vi "pulmonarytesting_pressurediameterlogging.vi"() -> ()   [LabVIEW 2014]
uses:
  <vilib>/vision/NI_Vision_Development_Module.lvlib
  <instrlib>/KD Scientific 2XX Series/KD Scientific 2XX Series.lvlib
panel:
  in  "stop 4":bool
  in  "Baud Rate (9600)":u32(ring)=9600 items=["300"=300, "1200"=1200, "2400"=2400, "4800"=4800, "9600"=9600]
  in  "Withdrawal Settings":T1={"Flow Rate (5)"=5.0, "Volume (10)"=10.0, "Volume Units (ml)"=enum."milliliters (ml)", "Rate Units (ml/min.)"=enum."milliliters per minute (ml/min.)"} {"Volume (10)" format="%#.3g"}
  in  "Diameter (8.75 mm)":dbl=8.75
  in  "Infusion Settings":T1={"Flow Rate (5)"=5.0, "Volume (10)"=10.0, "Volume Units (ml)"=enum."milliliters (ml)", "Rate Units (ml/min.)"=enum."milliliters per minute (ml/min.)"}
  out "Status":T2
  in  "stop 2":bool
  out "Delivered Volume":dbl
  out "Units":string
  in  "Operation Mode (Infuse)":u16(ring) items=["Infuse", "Withdraw", "Infuse-Withdraw", "Withdraw-Infuse", "Continuous"]
  in  "Address (0)":i32 format="%0.0f"
  in  "error in (no error)":errorcluster
  in  "VISA resource name":refnum<visa-resource-name>="COM1"
  in  "stop":bool
  out "Image":T3(plugin-control)
  out "Particle Measurements (Pixels) (Particle Analysis 1)":dbl[][](array[numeric]) format="%.2f"
  out "subarray":dbl[](array[numeric])
  out "The diameter":dbl[](array[numeric])
  in  "stop (F)":bool
  out "Data from Transducer":dynamicdata(graph) caption="Voltage from Transducer V"
  out "Voltage from pressure transducer":dbl[](array[numeric])
  out "Pressure mm Hg":dbl[](graph)
  in  "Calibration factor":dbl[](array[numeric])
  in  "Zero Error":dbl[](array[numeric])
  out "pressure mm Hg":dbl[](array[numeric])
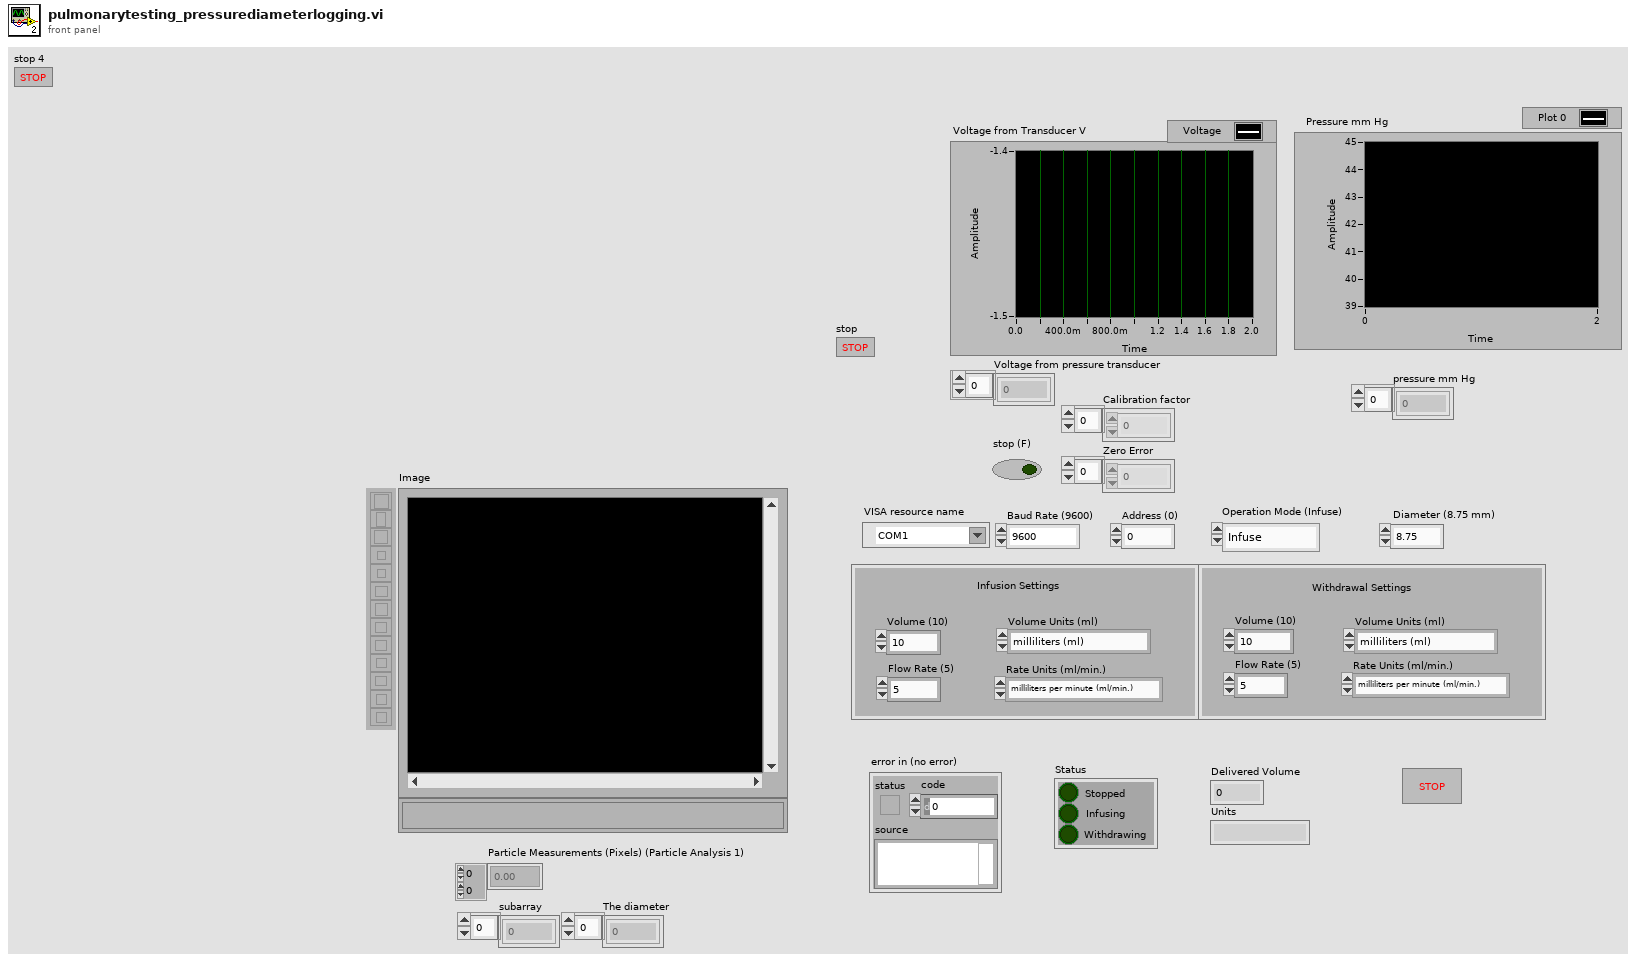
[diagram p1: front panel]
types:
  T1 = cluster{"Flow Rate (5)":dbl, "Volume (10)":dbl, "Volume Units (ml)":enum16{"milliliters (ml)", "microliters (ul)"}, "Rate Units (ml/min.)":enum16{"milliliters per minute (ml/min.)", "milliliters per hour (ml/hr.)", "microliters per minute (ul/min.)", "microliters per hour (ul/hr.)"}}
  T2 = cluster{"Stopped":bool, "Infusing":bool, "Withdrawing":bool}
  T3 = typedef "IMAQ Image.ctl" = refnum<image>
  T4 = typedef "Board Id" = u8
  T5 = typedef "ROI Descriptor" = cluster{"Global Rectangle":i32[], "Contours":cluster{"ID":enum32{"External", "Internal"}, "Type":u32, "Coordinates":i32[]}[]}
  T6 = enum16{"milliliters per minute (ml/min.)", "milliliters per hour (ml/hr.)", "microliters per minute (ul/min.)", "microliters per hour (ul/hr.)"}
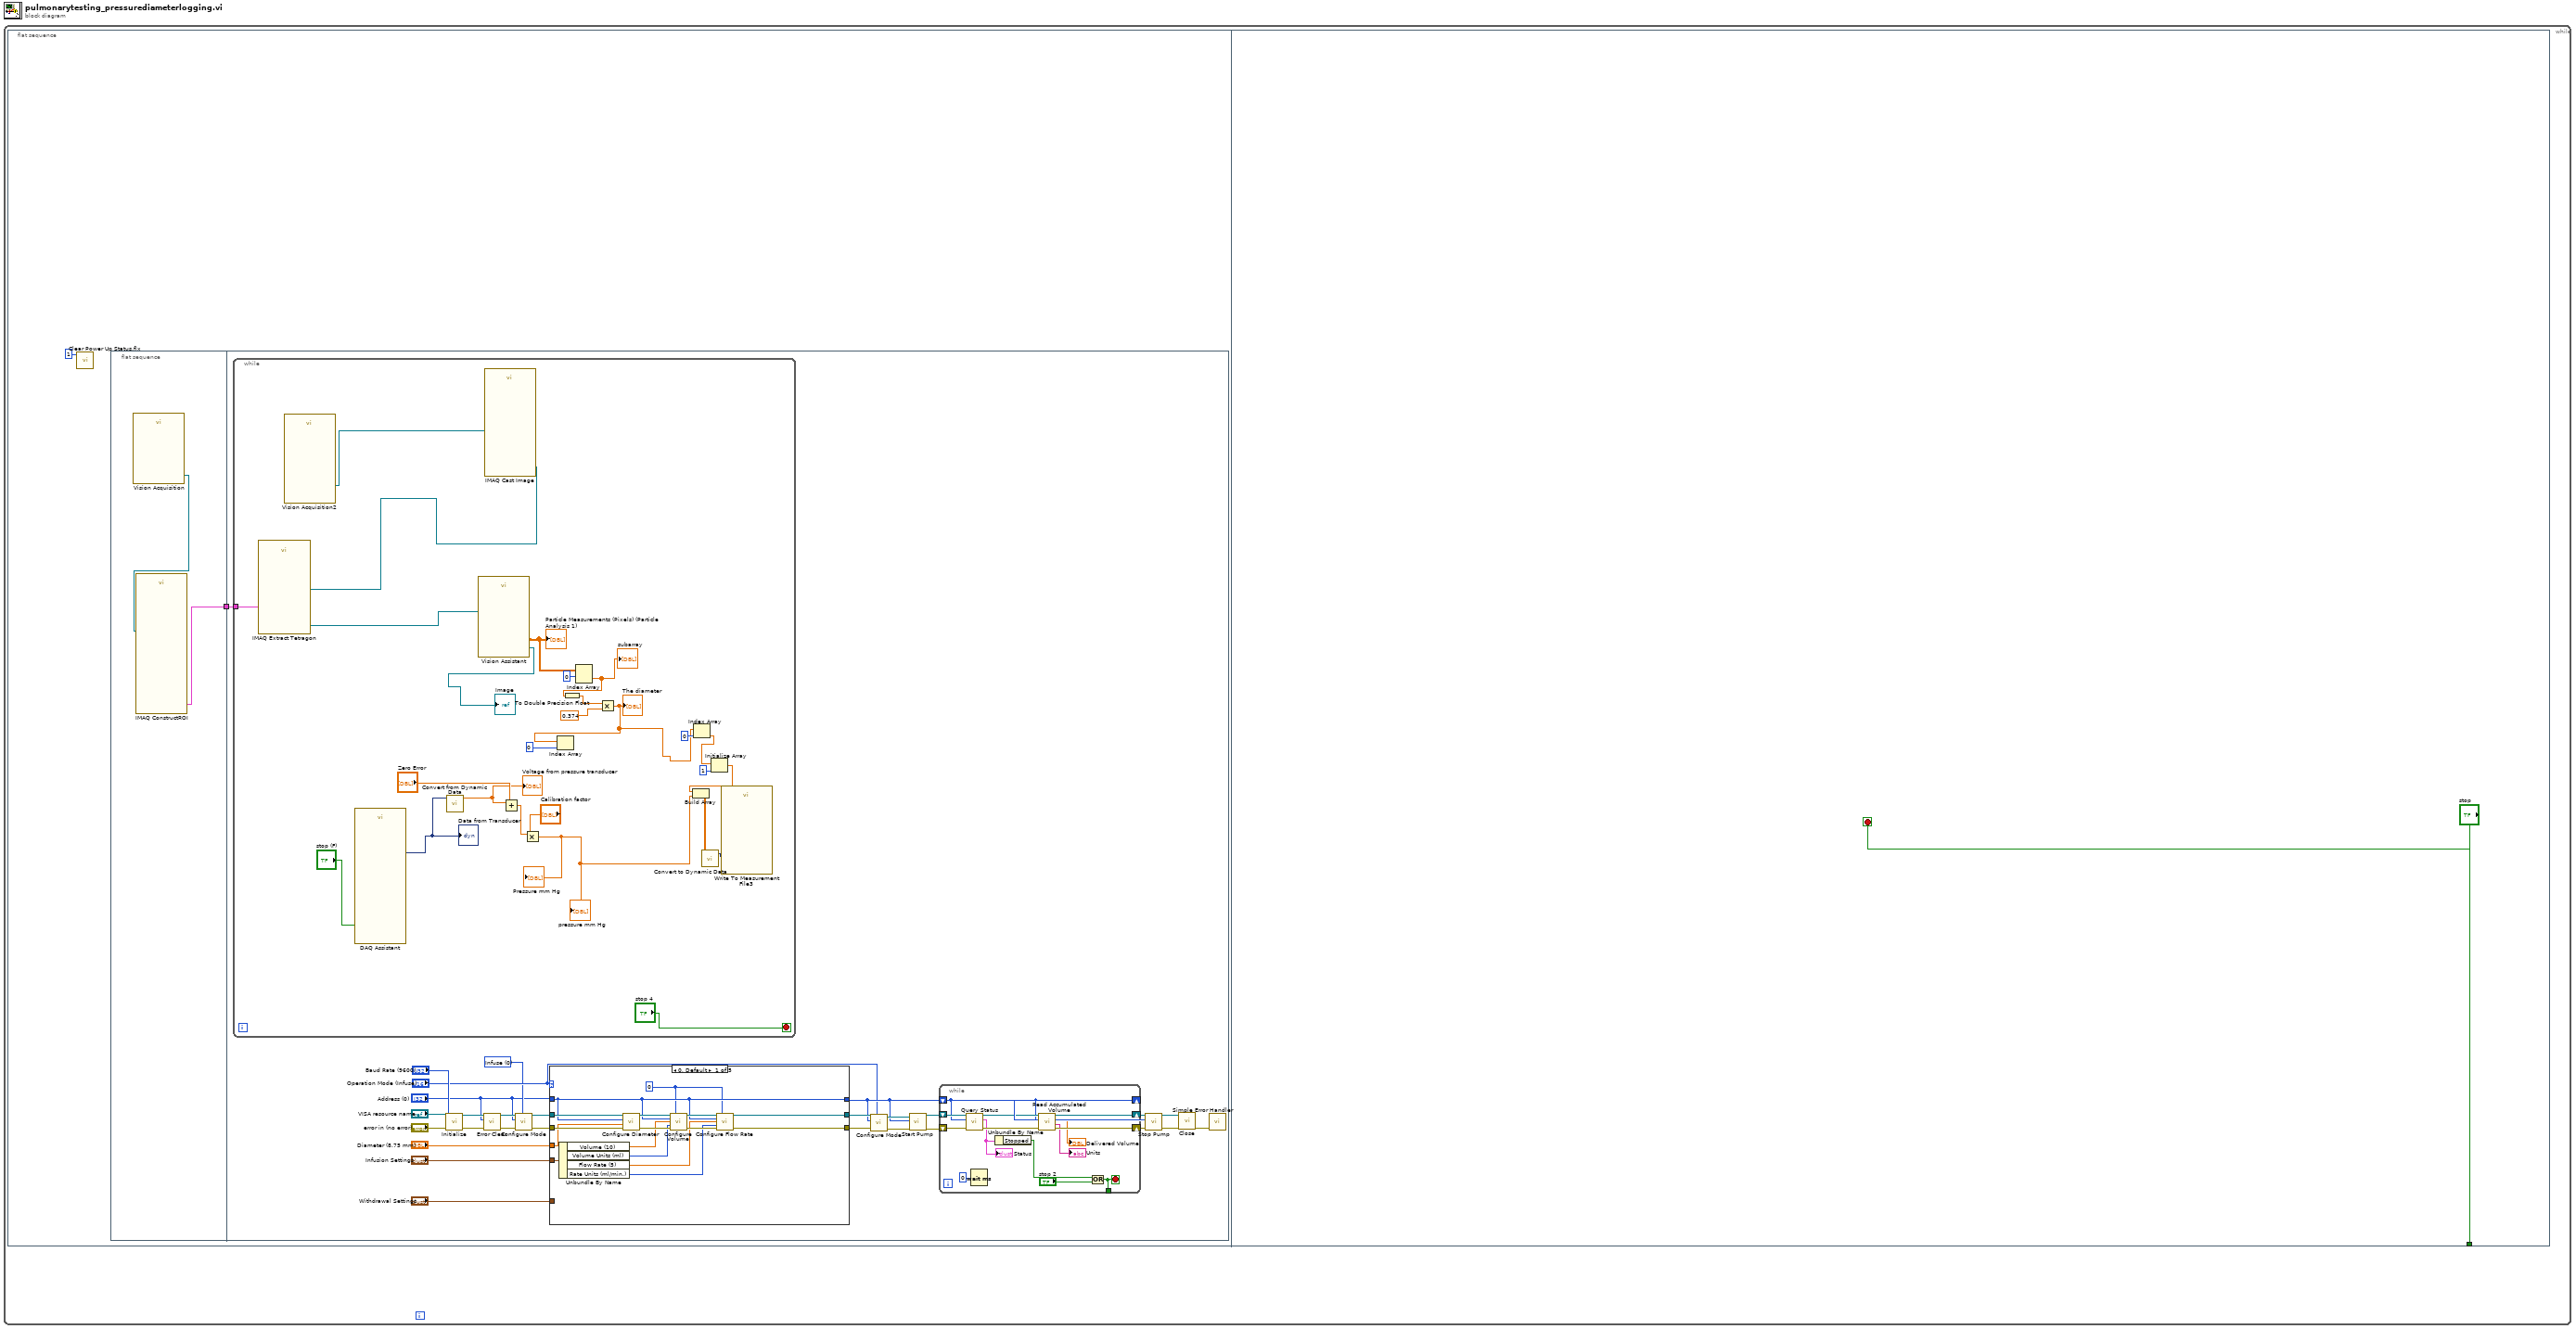
[diagram p0: block diagram]
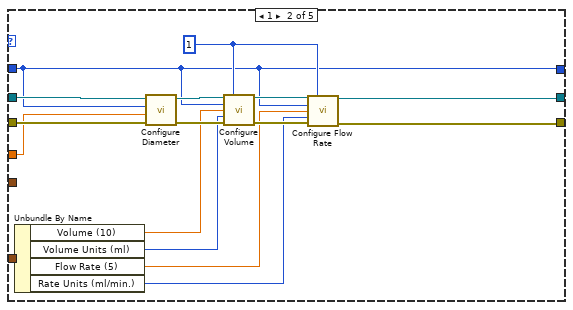
[diagram p2: hidden frame]
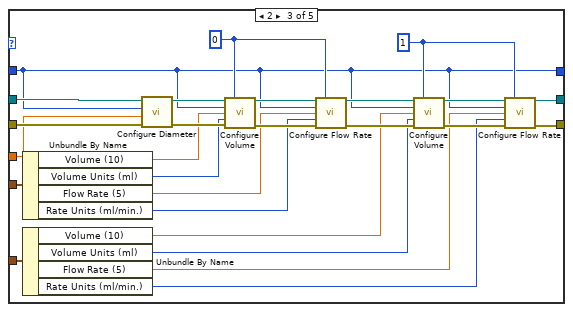
[diagram p3: hidden frame]
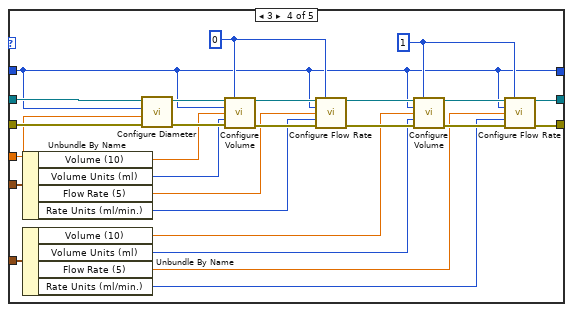
[diagram p4: hidden frame]
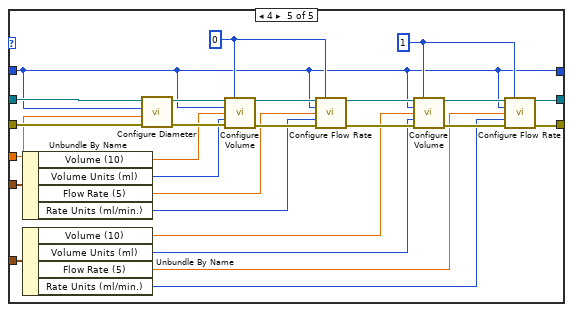
[diagram p5: hidden frame]
diagram:
  n1 = while {
    stop <- w1 stop-if-true
    n2 = flat-sequence {
      tunnel: ["stop"] -> w1
      frame #0 {
        n3 = call <vilib>:"Clear Power Up Status.flx"("Board ID"=T4 1) -> ()  [unwired: 6 in, 2 out]
        n4 = flat-sequence {
          tunnel: [w4] -> w3
          tunnel: w3 -> [w34]
          frame #0 {
            n5 = call "Vision Acquisition"() -> ("Image Out"=w5:T3)  [unwired: 26 in, 1 out]
            n6 = call "IMAQ ConstructROI"("Image"=w5) -> ("ROI Descriptor Out"=w4:T5)  [unwired: 7 in, 3 out]
          }
          frame #1 {
            w11 = u16 0 items=["Infuse", "Withdraw", "Infuse-Withdraw", "Withdraw-Infuse", "Continuous"] ("Mode (infuse)")
            n7 = while {
              tunnel: w34 -> [w60]
              stop <- "stop 4" stop-if-true
              n8 = call "Vision Acquisition2"() -> ("Image Out"=w44:T3)  [unwired: 25 in, 2 out]
              n9 = call "DAQ Assistant"("stop (F)"="stop (F)") -> ("data"=w59:dynamicdata)  [unwired: 15 in, 3 out]
              "Data from Transducer" <- w59
              n10 = call "Convert from Dynamic Data"("Dynamic Data Type"=w59) -> ("Array"=w56:dbl[])  [unwired: 3 in]
              "Voltage from pressure transducer" <- w56
              n11 = call "IMAQ Cast Image"("Image Src"=w44) -> ("Image Dst Out"=w51:T3)  [unwired: 9 in, 1 out]
              n12 = call-poly "IMAQ Extract Tetragon"("ROI Descriptor"=w60, "Image Src"=w51) -> ("Image Dst Out"=w52:T3)  [unwired: 8 in, 1 out]
              n13 = call "Vision Assistant"("Image In"=w52) -> ("Image Out"=→"Image":T3, "Particle Measurements (Pixels) (Particle Analysis 1)"=w50:dbl[][])  [unwired: 23 in, 2 out]
              "Particle Measurements (Pixels) (Particle Analysis 1)" <- w50
              n14 = Add(x=w56, y="Zero Error") -> (x+y=w58:dbl[])
              n15 = Multiply(x=w58, y="Calibration factor") -> (x*y=w42:dbl[])
              "Pressure mm Hg" <- w42
              "pressure mm Hg" <- w42
              n16 = Index Array(array=w50, index (row)=0) -> (element=w48:dbl[])  [unwired: 1 in]
              "subarray" <- w48
              n17 = To Double Precision Float(number=w48) -> (double precision float=w47:dbl[])
              n18 = Multiply(x=w47, y=0.374) -> (x*y=w40:dbl[])
              "The diameter" <- w40
              n19 = Index Array(array=w40, index=0) -> ()  [unwired: 1 out]
              n20 = Index Array(array=w40, index=0) -> (element=w39:dbl)
              n21 = Initialize Array(w39, 1 ("dimension size")) -> (w37:dbl[])
              n22 = Build Array(w37, w42) -> (w36:dbl[][])
              n23 = call "Convert to Dynamic Data"("2D Array"=w36) -> ("Dynamic Data Type"=w35:dynamicdata)  [unwired: 3 in]
              n24 = call "Write To Measurement File3"("Signals"=w35) -> ()  [unwired: 16 in, 3 out]
            }
            n25 = call <instrlib>:"Initialize.vi"("error in (no error)"="error in (no error)", "Baud Rate (9600)"="Baud Rate (9600)", "VISA resource name"="VISA resource name") -> ("error out"=w8:errorcluster, "VISA resource name out"=w7:refnum<visa-resource-name>)  [unwired: 7 in]
            n26 = call <instrlib>:"Error Clear.vi"("error in (no error)"=w8, "Address (0)"="Address (0)", "VISA resource name"=w7) -> ("error out"=w9:errorcluster, "VISA resource name out"=w10:refnum<visa-resource-name>)  [unwired: 6 in, 1 out]
            n27 = call <instrlib>:"Configure Mode.vi"("Mode (infuse)"=w11, "error in (no error)"=w9, "Address (0)"="Address (0)", "VISA resource name"=w10) -> ("error out"=w13:errorcluster, "VISA resource name out"=w12:refnum<visa-resource-name>)  [unwired: 6 in]
            n28 = case shown="0, Default" "Operation Mode (Infuse)" {
              tunnel: "Infusion Settings" -> [w70 _ w118 w144 w170]
              tunnel: "Withdrawal Settings" -> [_ w92 w117 w143 w169]
              tunnel: w12 -> [w76 w91 w116 w142 w168]
              tunnel: w13 -> [w75 w87 w115 w141 w167]
              tunnel: "Diameter (8.75 mm)" -> [w69 w83 w98 w124 w150]
              tunnel: [w68 w77 w93 w119 w145] -> w15
              tunnel: "Address (0)" -> [w68 w77 w93 w119 w145]
              tunnel: [w63 w88 w95 w121 w147] -> w19
              tunnel: [w62 w84 w94 w120 w146] -> w18
              frame 0, Default {
                w61 = 0
                n29 = Unbundle By Name(w70) -> ("Volume (10)"=w67:dbl, "Volume Units (ml)"=w66:enum16{"milliliters (ml)", "microliters (ul)"}, "Flow Rate (5)"=w65:dbl, "Rate Units (ml/min.)"=w64:T6)
                n30 = call <instrlib>:"Configure Diameter.vi"("error in (no error)"=w75, "Diameter (8.75 mm)"=w69, "Address (0)"=w68, "VISA resource name"=w76) -> ("error out"=w73:errorcluster, "VISA resource name out"=w74:refnum<visa-resource-name>)  [unwired: 6 in]
                n31 = call <instrlib>:"Configure Volume.vi"("VISA resource name"=w74, "Mode (infuse)"=w61, "Address (0)"=w68, "Volume (100)"=w67, "Units (0: milliliters)"=w66, "error in (no error)"=w73) -> ("VISA resource name out"=w72:refnum<visa-resource-name>, "error out"=w71:errorcluster)  [unwired: 8 in]
                n32 = call <instrlib>:"Configure Flow Rate.vi"("VISA resource name"=w72, "Mode (infuse)"=w61, "Address (0)"=w68, "Flow Rate (5)"=w65, "Units (0: milliliters per minute)"=w64, "error in (no error)"=w71) -> ("VISA resource name out"=w63:refnum<visa-resource-name>, "error out"=w62:errorcluster)  [unwired: 8 in]
              }
              frame 1 {
                w78 = 1
                n33 = Unbundle By Name(w92) -> ("Volume (10)"=w82:dbl, "Volume Units (ml)"=w81:enum16{"milliliters (ml)", "microliters (ul)"}, "Flow Rate (5)"=w80:dbl, "Rate Units (ml/min.)"=w79:T6)
                n34 = call <instrlib>:"Configure Diameter.vi"("error in (no error)"=w87, "Diameter (8.75 mm)"=w83, "Address (0)"=w77, "VISA resource name"=w91) -> ("error out"=w86:errorcluster, "VISA resource name out"=w90:refnum<visa-resource-name>)  [unwired: 6 in]
                n35 = call <instrlib>:"Configure Volume.vi"("VISA resource name"=w90, "Mode (infuse)"=w78, "Address (0)"=w77, "Volume (100)"=w82, "Units (0: milliliters)"=w81, "error in (no error)"=w86) -> ("VISA resource name out"=w89:refnum<visa-resource-name>, "error out"=w85:errorcluster)  [unwired: 8 in]
                n36 = call <instrlib>:"Configure Flow Rate.vi"("VISA resource name"=w89, "Mode (infuse)"=w78, "Address (0)"=w77, "Flow Rate (5)"=w80, "Units (0: milliliters per minute)"=w79, "error in (no error)"=w85) -> ("VISA resource name out"=w88:refnum<visa-resource-name>, "error out"=w84:errorcluster)  [unwired: 8 in]
              }
              frame 2 {
                w96 = 1
                w97 = 0
                n37 = Unbundle By Name(w118) -> ("Volume (10)"=w106:dbl, "Volume Units (ml)"=w105:enum16{"milliliters (ml)", "microliters (ul)"}, "Flow Rate (5)"=w104:dbl, "Rate Units (ml/min.)"=w103:T6)
                n38 = Unbundle By Name(w117) -> ("Volume (10)"=w102:dbl, "Volume Units (ml)"=w101:enum16{"milliliters (ml)", "microliters (ul)"}, "Flow Rate (5)"=w100:dbl, "Rate Units (ml/min.)"=w99:T6)
                n39 = call <instrlib>:"Configure Diameter.vi"("error in (no error)"=w115, "Diameter (8.75 mm)"=w98, "Address (0)"=w93, "VISA resource name"=w116) -> ("error out"=w110:errorcluster, "VISA resource name out"=w114:refnum<visa-resource-name>)  [unwired: 6 in]
                n40 = call <instrlib>:"Configure Volume.vi"("VISA resource name"=w114, "Mode (infuse)"=w97, "Address (0)"=w93, "Volume (100)"=w106, "Units (0: milliliters)"=w105, "error in (no error)"=w110) -> ("VISA resource name out"=w113:refnum<visa-resource-name>, "error out"=w109:errorcluster)  [unwired: 8 in]
                n41 = call <instrlib>:"Configure Flow Rate.vi"("VISA resource name"=w113, "Mode (infuse)"=w97, "Address (0)"=w93, "Flow Rate (5)"=w104, "Units (0: milliliters per minute)"=w103, "error in (no error)"=w109) -> ("VISA resource name out"=w112:refnum<visa-resource-name>, "error out"=w108:errorcluster)  [unwired: 8 in]
                n42 = call <instrlib>:"Configure Volume.vi"("VISA resource name"=w112, "Mode (infuse)"=w96, "Address (0)"=w93, "Volume (100)"=w102, "Units (0: milliliters)"=w101, "error in (no error)"=w108) -> ("VISA resource name out"=w111:refnum<visa-resource-name>, "error out"=w107:errorcluster)  [unwired: 8 in]
                n43 = call <instrlib>:"Configure Flow Rate.vi"("VISA resource name"=w111, "Mode (infuse)"=w96, "Address (0)"=w93, "Flow Rate (5)"=w100, "Units (0: milliliters per minute)"=w99, "error in (no error)"=w107) -> ("VISA resource name out"=w95:refnum<visa-resource-name>, "error out"=w94:errorcluster)  [unwired: 8 in]
              }
              frame 3 {
                w122 = 1
                w123 = 0
                n44 = Unbundle By Name(w144) -> ("Volume (10)"=w132:dbl, "Volume Units (ml)"=w131:enum16{"milliliters (ml)", "microliters (ul)"}, "Flow Rate (5)"=w130:dbl, "Rate Units (ml/min.)"=w129:T6)
                n45 = Unbundle By Name(w143) -> ("Volume (10)"=w128:dbl, "Volume Units (ml)"=w127:enum16{"milliliters (ml)", "microliters (ul)"}, "Flow Rate (5)"=w126:dbl, "Rate Units (ml/min.)"=w125:T6)
                n46 = call <instrlib>:"Configure Diameter.vi"("error in (no error)"=w141, "Diameter (8.75 mm)"=w124, "Address (0)"=w119, "VISA resource name"=w142) -> ("error out"=w136:errorcluster, "VISA resource name out"=w140:refnum<visa-resource-name>)  [unwired: 6 in]
                n47 = call <instrlib>:"Configure Volume.vi"("VISA resource name"=w140, "Mode (infuse)"=w123, "Address (0)"=w119, "Volume (100)"=w132, "Units (0: milliliters)"=w131, "error in (no error)"=w136) -> ("VISA resource name out"=w139:refnum<visa-resource-name>, "error out"=w135:errorcluster)  [unwired: 8 in]
                n48 = call <instrlib>:"Configure Flow Rate.vi"("VISA resource name"=w139, "Mode (infuse)"=w123, "Address (0)"=w119, "Flow Rate (5)"=w130, "Units (0: milliliters per minute)"=w129, "error in (no error)"=w135) -> ("VISA resource name out"=w138:refnum<visa-resource-name>, "error out"=w134:errorcluster)  [unwired: 8 in]
                n49 = call <instrlib>:"Configure Volume.vi"("VISA resource name"=w138, "Mode (infuse)"=w122, "Address (0)"=w119, "Volume (100)"=w128, "Units (0: milliliters)"=w127, "error in (no error)"=w134) -> ("VISA resource name out"=w137:refnum<visa-resource-name>, "error out"=w133:errorcluster)  [unwired: 8 in]
                n50 = call <instrlib>:"Configure Flow Rate.vi"("VISA resource name"=w137, "Mode (infuse)"=w122, "Address (0)"=w119, "Flow Rate (5)"=w126, "Units (0: milliliters per minute)"=w125, "error in (no error)"=w133) -> ("VISA resource name out"=w121:refnum<visa-resource-name>, "error out"=w120:errorcluster)  [unwired: 8 in]
              }
              frame 4 {
                w148 = 1
                w149 = 0
                n51 = Unbundle By Name(w170) -> ("Volume (10)"=w158:dbl, "Volume Units (ml)"=w157:enum16{"milliliters (ml)", "microliters (ul)"}, "Flow Rate (5)"=w156:dbl, "Rate Units (ml/min.)"=w155:T6)
                n52 = Unbundle By Name(w169) -> ("Volume (10)"=w154:dbl, "Volume Units (ml)"=w153:enum16{"milliliters (ml)", "microliters (ul)"}, "Flow Rate (5)"=w152:dbl, "Rate Units (ml/min.)"=w151:T6)
                n53 = call <instrlib>:"Configure Diameter.vi"("error in (no error)"=w167, "Diameter (8.75 mm)"=w150, "Address (0)"=w145, "VISA resource name"=w168) -> ("error out"=w162:errorcluster, "VISA resource name out"=w166:refnum<visa-resource-name>)  [unwired: 6 in]
                n54 = call <instrlib>:"Configure Volume.vi"("VISA resource name"=w166, "Mode (infuse)"=w149, "Address (0)"=w145, "Volume (100)"=w158, "Units (0: milliliters)"=w157, "error in (no error)"=w162) -> ("VISA resource name out"=w165:refnum<visa-resource-name>, "error out"=w161:errorcluster)  [unwired: 8 in]
                n55 = call <instrlib>:"Configure Flow Rate.vi"("VISA resource name"=w165, "Mode (infuse)"=w149, "Address (0)"=w145, "Flow Rate (5)"=w156, "Units (0: milliliters per minute)"=w155, "error in (no error)"=w161) -> ("VISA resource name out"=w164:refnum<visa-resource-name>, "error out"=w160:errorcluster)  [unwired: 8 in]
                n56 = call <instrlib>:"Configure Volume.vi"("VISA resource name"=w164, "Mode (infuse)"=w148, "Address (0)"=w145, "Volume (100)"=w154, "Units (0: milliliters)"=w153, "error in (no error)"=w160) -> ("VISA resource name out"=w163:refnum<visa-resource-name>, "error out"=w159:errorcluster)  [unwired: 8 in]
                n57 = call <instrlib>:"Configure Flow Rate.vi"("VISA resource name"=w163, "Mode (infuse)"=w148, "Address (0)"=w145, "Flow Rate (5)"=w152, "Units (0: milliliters per minute)"=w151, "error in (no error)"=w159) -> ("VISA resource name out"=w147:refnum<visa-resource-name>, "error out"=w146:errorcluster)  [unwired: 8 in]
              }
            }
            n58 = call <instrlib>:"Configure Mode.vi"("Mode (infuse)"="Operation Mode (Infuse)", "error in (no error)"=w18, "Address (0)"=w15, "VISA resource name"=w19) -> ("error out"=w16:errorcluster, "VISA resource name out"=w17:refnum<visa-resource-name>)  [unwired: 6 in]
            n59 = call <instrlib>:"Start Pump.vi"("error in (no error)"=w16, "Address (0)"=w15, "VISA resource name"=w17) -> ("error out"=w30:errorcluster, "VISA resource name out"=w31:refnum<visa-resource-name>)  [unwired: 7 in]
            n60 = while {
              shift-right: [w174] -> w24
              shift-left: w15 -> [w174]
              shift-right: [w176] -> w29
              shift-left: w31 -> [w181]
              shift-right: [w175] -> w28
              shift-left: w30 -> [w182]
              tunnel: [w171] -> _
              stop <- w171 stop-if-true
              n61 = call <instrlib>:"Query Status.vi"("error in (no error)"=w182, "Address (0)"=w174, "VISA resource name"=w181) -> ("error out"=w184:errorcluster, "Status"=w180:T2, "VISA resource name out"=w177:refnum<visa-resource-name>)  [unwired: 6 in]
              "Status" <- w180
              n62 = Wait (ms)(milliseconds to wait=u32 0) -> ()  [unwired: 1 out]
              n63 = Unbundle By Name(w180) -> ("Stopped"=w179:bool)
              n64 = call <instrlib>:"Read Accumulated Volume.vi"("error in (no error)"=w184, "Address (0)"=w174, "VISA resource name"=w177) -> ("error out"=w175:errorcluster, "Units"=→"Units":string, "Delivered Volume"=→"Delivered Volume":dbl, "VISA resource name out"=w176:refnum<visa-resource-name>)  [unwired: 5 in]
              n65 = Or(x=w179, y="stop 2") -> (x .or. y?=w171:bool)
            }
            n66 = call <instrlib>:"Stop Pump.vi"("error in (no error)"=w28, "Address (0)"=w24, "VISA resource name"=w29) -> ("error out"=w22:errorcluster, "VISA resource name out"=w21:refnum<visa-resource-name>)  [unwired: 7 in]
            n67 = call <instrlib>:"Close.vi"("error in (no error)"=w22, "VISA resource name"=w21) -> ("error out"=w23:errorcluster)  [unwired: 9 in]
            n68 = call <vilib>:"Simple Error Handler.vi"("error in (no error)"=w23) -> ()  [unwired: 4 in, 5 out]
          }
        }
      }
      frame #1 {
      }
    }
  }
